vi "Handle Error.vi"(8 "error in (no error)":errorcluster, 11 "ErrorLog in":refnum<class "ErrorLog.lvclass">) -> (0 "error out":errorcluster, 2 "stop actor?":bool=TRUE, 3 "ErrorLog out":refnum<class "ErrorLog.lvclass">)   [LabVIEW 2019, in "ErrorLog.lvlib" / "ErrorLog.lvclass"]
doc: "(<B>Filename</B>: Actor Framework.lvlib:Actor.lvclass:Handle Error.vi)\n\nDefines how the actor handles an error that occurred while processing a message. By default, this method does nothing except stop the actor."
uses:
  ErrorLog.lvclass
  Classes/Error/Error.lvclass
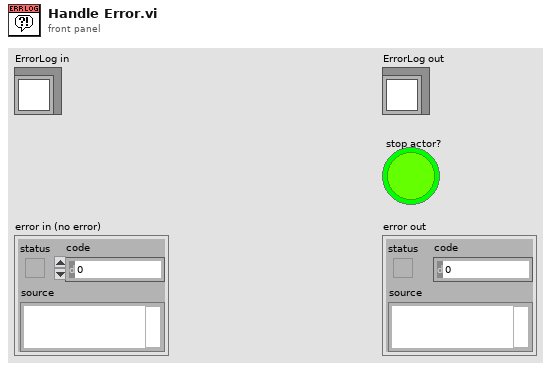
[diagram p1: front panel]
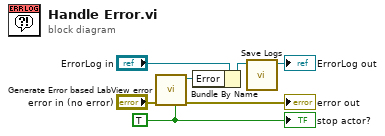
[diagram p0: block diagram]
diagram:
  w1 = TRUE ("Deactive Save Error?")
  n1 = call "Generate Error based LabView error.vi"("Deactive Save Error?"=w1, "Error In"="error in (no error)") -> ("Error Out"=→"error out":errorcluster, "Error"=w5:refnum<class "Error.lvclass">)  [unwired: 8 in]
  n2 = Bundle By Name(cluster="ErrorLog in", "Error"=w5) -> (w4:refnum<class "ErrorLog.lvclass">)
  n3 = call-dynamic "Save Logs.vi"("EventLog in"=w4) -> ("EventLog out"=→"ErrorLog out":refnum<class "ErrorLog.lvclass">)  [unwired: 9 in, 1 out]
  "stop actor?" <- w1
